vi "Maestro.vi"() -> ()   [LabVIEW 2017]
panel:
  in  "300001":u16
  out "000001":bool
  out "000002":u16
  in  "stop":bool
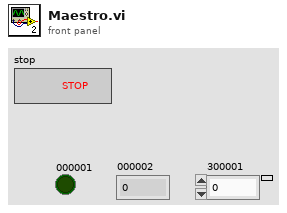
[diagram p1: front panel]
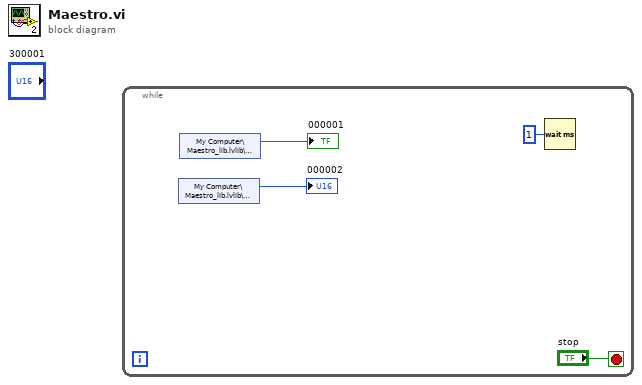
[diagram p0: block diagram]
diagram:
  n1 = while {
    stop <- "stop" stop-if-true
    n2 = shared-variable "My Computer\\Maestro_lib.lvlib\\000002"() -> (→"000002":u16)  [unwired: 1 in, 1 out]
    n3 = shared-variable "My Computer\\Maestro_lib.lvlib\\000001"() -> (→"000001":bool)  [unwired: 1 in, 1 out]
    n4 = Wait (ms)(milliseconds to wait=u32 1) -> ()  [unwired: 1 out]
  }
